vi "字符转浮点数.vi"(9 "十六进制32bit":string) -> (1 "数值":sgl)   [LabVIEW 2020]
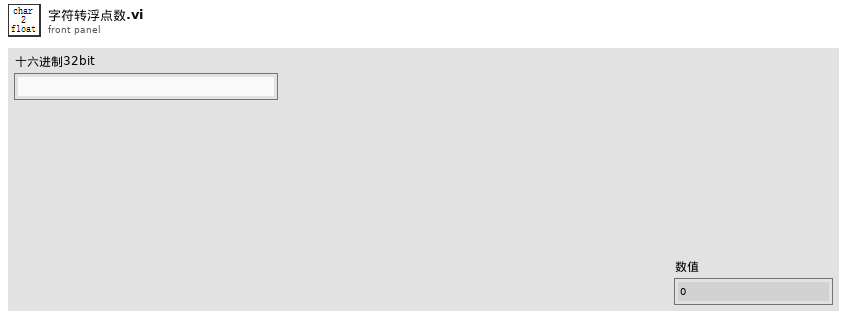
[diagram p1: front panel]
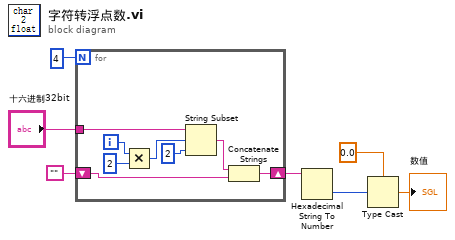
[diagram p0: block diagram]
diagram:
  n1 = for {
    N: 4 -> [_]
    tunnel: "十六进制32bit" -> [w14]
    shift-right: [w13] -> w2
    shift-left: "" -> [w12]
    i -> [w10]
    n2 = Multiply(x=w10, y=2 ("长度（剩余）")) -> (x*y=w9:i32)
    n3 = String Subset(string=w14, offset (0)=w9, length (rest)=2 ("长度（剩余）")) -> (substring=w11:string)
    n4 = Concatenate Strings(w11, w12) -> (w13:string)
  }
  n5 = Hexadecimal String To Number(string=w2) -> (number=w1:u32)  [unwired: 2 in, 1 out]
  n6 = Type Cast(type=sgl 0.0, x=w1) -> (*(type *) &x=→"数值":sgl)
